vi "Performance test.vi"() -> ()   [LabVIEW 8.6]
panel:
  in  "deviceId":i32
  in  "Path to LUT file":path=path "C:/BLINK_PCIe/LUT_Files/linear.lut"
  out "XY Graph":cluster{i32[], dbl[]}(graph)
  out "Current number of spots":i32=100
  out "Current execution time":dbl=38.0
  in  "alpha RPC":sgl=1.0
  in  "Number of spotsmax":i32=100
  in  "Number of spots min":i32=1
  in  "TrueFrame":i32=3
  in  "Number of \ntime to execute":i32=10
  in  "stop program":bool
  out "Generated Hologram":u8[][](graph)
  in  "method":i32=1
  in  "N_iterations":i32=10
  in  "SLM enabled":bool
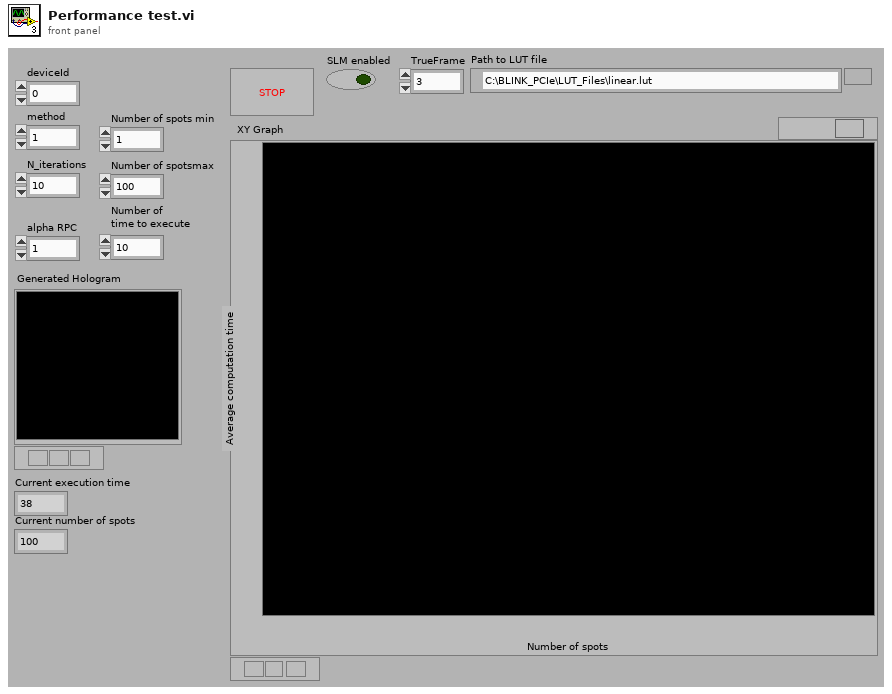
[diagram p1: front panel]
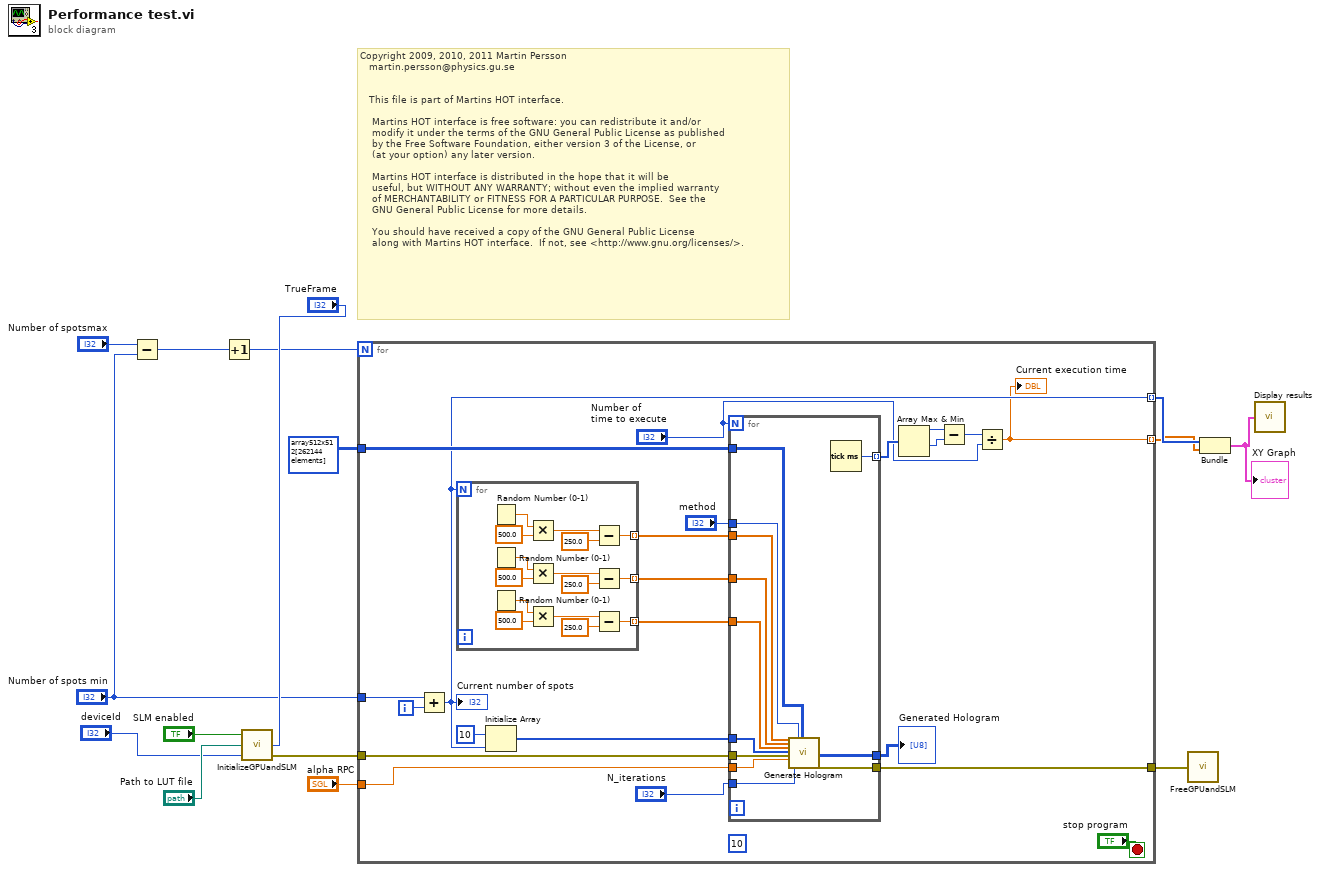
[diagram p0: block diagram]
diagram:
  # "Copyright 2009, 2010, 2011 Martin Persson \n   martin.persson@physics.gu.se\n\n\n   This file is part of Martins HOT interface.\n\n    Martins HOT interface is free software: you can redistribute it and/or \n    modify it under the terms of the GNU General Public License as published \n    by the Free Software Foundation, either version 3 of the License, or\n    (at your option) any later version.\n\n    Martins HOT interface is distributed in the hope that it will be \n    useful, but WITHOUT ANY WARRANTY; without even the implied warranty\n    of MERCHANTABILITY or FITNESS FOR A PARTICULAR PURPOSE.  See the\n    GNU General Public License for more details.\n\n    You should have received a copy of the GNU General Public License\n    along with Martins HOT interface.  If not, see <http://www.gnu.org/licenses/>."
  n1 = Subtract(x="Number of spotsmax", y="Number of spots min") -> (x-y=w10:i32)
  n2 = Increment(x=w10) -> (x+1=w8:i32)
  n3 = call "InitializeGPUandSLM.vi"("TrueFrame"="TrueFrame", "deviceId"="deviceId", "Path to LUT file"="Path to LUT file", "SLM enabled"="SLM enabled") -> ("CUDA/SLM error"=w14:errorcluster)  [unwired: 1 out]
  n4 = for {
    N: w8 -> [_]
    tunnel: w14 -> [w37]
    tunnel: [w34] -> w13
    tunnel: u8[][] array512x512[262144 elements] ("Default") -> [w32]
    tunnel: "Number of spots min" -> [w24]
    tunnel: [w16] -> w3 mode=indexing
    tunnel: [w17] -> w4 mode=indexing
    tunnel: "alpha RPC" -> [w19]
    i -> [w23]
    stop <- "stop program" stop-if-true
    (unwired) 10 ("element")
    n5 = Add(x=w24, y=w23) -> (x+y=w17:i32)
    "Current number of spots" <- w17
    n6 = for {
      N: w17 -> [_]
      tunnel: [w41] -> w22 mode=indexing
      tunnel: [w40] -> w21 mode=indexing
      tunnel: [w39] -> w20 mode=indexing
      n7 = Random Number (0-1)() -> (number: 0 to 1=w52:dbl)
      n8 = Random Number (0-1)() -> (number: 0 to 1=w45:dbl)
      n9 = Random Number (0-1)() -> (number: 0 to 1=w38:dbl)
      n10 = Multiply(x=w52, y=500.0) -> (x*y=w50:dbl)
      n11 = Multiply(x=w45, y=500.0) -> (x*y=w47:dbl)
      n12 = Multiply(x=w38, y=500.0) -> (x*y=w43:dbl)
      n13 = Subtract(x=w50, y=250.0) -> (x-y=w41:dbl)
      n14 = Subtract(x=w47, y=250.0) -> (x-y=w40:dbl)
      n15 = Subtract(x=w43, y=250.0) -> (x-y=w39:dbl)
    }
    n16 = Initialize Array(10 ("element"), w17) -> (w30:i32[])
    n17 = for {
      N: "Number of \ntime to execute" -> [_]
      tunnel: w37 -> [w64]
      tunnel: "N_iterations" -> [w63]
      tunnel: w21 -> [w62]
      tunnel: w20 -> [w61]
      tunnel: "method" -> [w60]
      tunnel: [w59] -> w34
      tunnel: [w58] -> w33
      tunnel: w32 -> [w57]
      tunnel: w22 -> [w56]
      tunnel: w30 -> [w55]
      tunnel: [w54] -> w29 mode=indexing
      tunnel: w19 -> [w53]
      n18 = call "Generate Hologram.vi"("x"=w56, "y"=w62, "z"=w61, "spot_intensities"=w55, "CUDA/SLM error in"=w64, "alpha RPC"=w53, "N_iterations"=w63, "method"=w60, "CGH in"=w57) -> ("CGH out"=w58:u8[][], "CUDA/SLM error out"=w59:errorcluster)  [unwired: 16 in, 1 out]
      n19 = Tick Count (ms)() -> (millisecond timer value=w54:u32)
    }
    "Generated Hologram" <- w33
    n20 = Array Max & Min(array=w29) -> (max value=w28:u32, min value=w27:u32)  [unwired: 2 out]
    n21 = Subtract(x=w28, y=w27) -> (x-y=w26:u32)
    n22 = Divide(x=w26, y="Number of \ntime to execute") -> (x/y=w16:dbl)
    "Current execution time" <- w16
  }
  n23 = call "FreeGPUandSLM.vi"("error in"=w13) -> ()  [unwired: 1 out]
  n24 = Bundle(w4, w3) -> (w2:cluster{i32[], dbl[]})  [unwired: 1 in]
  "XY Graph" <- w2
  n25 = call "Display results.vi"("Cluster"=w2) -> ()
